vi "tb_real sequence extract.vi"() -> ()   [LabVIEW 2011]
uses:
  <userlib>/FPGA Library/Code Development/Signal Processing/FFT Block/FFT/FFT Size.ctl
  <vilib>/rvi/FXPMathLib/FxpInterpret/XNode/nifxpmath_Interpret.xnode
panel:
  in  "stop":bool
  out "Iterations":i32
  out "Imag":dbl[](array[numeric])
  out "Real":dbl[](array[numeric])
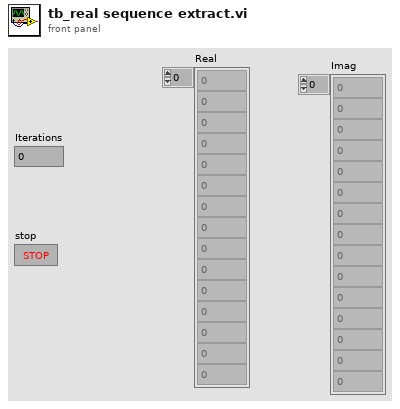
[diagram p1: front panel]
types:
  T1 = typedef "FFT Size.ctl" = enum16{"32", "64", "128", "256", "512", "1024", "2048", "4096", "8192", "16384", "32768", "65536"}
  T2 = cluster{"xk_im":fxp<+,32,32>, "xk_re":fxp<+,32,32>}
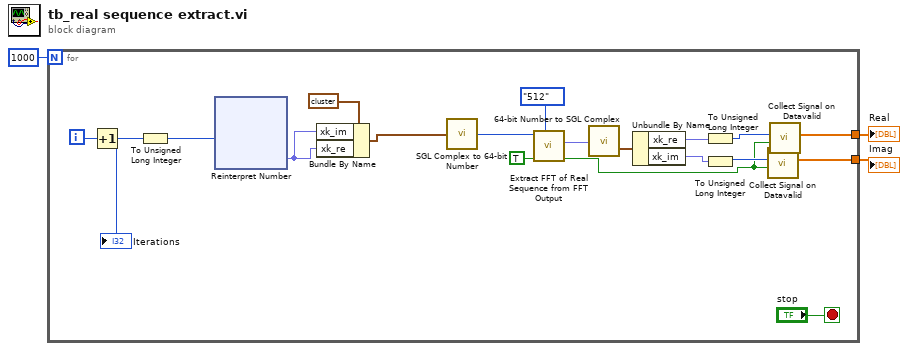
[diagram p0: block diagram]
diagram:
  n1 = for {
    N: 1000 -> [_]
    tunnel: [w14] -> w2
    tunnel: [w6] -> w1
    i -> [w20]
    stop <- "stop" stop-if-true
    n2 = Increment(x=w20) -> (x+1=w15:i32)
    n3 = To Unsigned Long Integer(number=w15) -> (unsigned 32bit integer=w19:u32)
    n4 = xnode "Reinterpret Number"("x"=w19) -> ("y"=w18:fxp<+,32,32>)
    n5 = Bundle By Name(cluster=T2 {"xk_im"=0.0, "xk_re"=0.0} ("Input CSG"), "xk_im"=w18, "xk_re"=w18) -> (w17:T2)
    n6 = call <userlib>:"SGL Complex to 64-bit Number.vi"("Input CSG"=w17) -> ("64-bit Complex"=w22:u64)  [unwired: 14 in]
    n7 = call <userlib>:"Extract FFT of Real Sequence from FFT Output.vi"("FFT Size"=FFT_Size."512", "Input Valid"=TRUE, "Input X(k)"=w22) -> ("Output Valid"=w7:bool, "X(N-k)"=w13:fxp<+,64,64>)  [unwired: 6 in, 1 out]
    n8 = call <userlib>:"64-bit Number to SGL Complex.vi"("Input"=w13) -> ("Complex Number"=w12:T2)  [unwired: 14 in]
    n9 = Unbundle By Name(w12) -> ("xk_re"=w11:fxp<+,32,32>, "xk_im"=w10:fxp<+,32,32>)
    n10 = To Unsigned Long Integer(number=w11) -> (unsigned 32bit integer=w9:u32)
    n11 = To Unsigned Long Integer(number=w10) -> (unsigned 32bit integer=w8:u32)
    n12 = call <userlib>:"Collect Signal on Datavalid.vi"("Data Valid"=w7, "Input"=w8) -> ("Output"=w6:dbl[])  [unwired: 9 in]
    n13 = call <userlib>:"Collect Signal on Datavalid.vi"("Data Valid"=w7, "Input"=w9) -> ("Output"=w14:dbl[])  [unwired: 9 in]
    "Iterations" <- w20
  }
  "Real" <- w2
  "Imag" <- w1
